vi "Acq_N_Proc.vi"(0 "I2C Ref In":T1={"myRIO Reference"={"myRIO Model"=enum."Unknown", "myRIO Hardware Reference"={"Generic FPGA Reference"=refnum, "Allow multiple opens"=FALSE}}, "I2C Channels Enum"=enum."Not Connected", "I2C Configuration"={"I2C Transfer Rate"=enum."Fast mode (400 kbps)"}}, 1 "Slave_Adress":u8 format="%02o", 2 "I2C Errors":errorcluster, 4 "DIO Ref In":T9, 5 "Int Errors":errorcluster) -> (19 "error IO":errorcluster)   [LabVIEW 2014]
uses:
  <vilib>/myRIO/Instrument Drivers/Onboard IO/DIO/typedefs/DIO Reference.ctl
  <vilib>/myRIO/Common/Instrument Driver Framework/Utilities/typedefs/myRIO Generic Hardware Reference.ctl
  <vilib>/myRIO/Common/Instrument Driver Framework/Utilities/typedefs/Hardware Version Enum.ctl
  <vilib>/myRIO/Common/Instrument Driver Framework/Utilities/typedefs/myRIO v1.0 Reference.ctl
  <vilib>/myRIO/Common/Instrument Driver Framework/Utilities/typedefs/Generic FPGA Reference.ctl
  <vilib>/myRIO/Common/Instrument Driver Framework/myRIO v1.0/DIO/typedefs/DIO Channels List.ctl
  <vilib>/myRIO/Common/Instrument Driver Framework/myRIO v1.0/DIO/typedefs/DIO Channels Enum.ctl
  <vilib>/myRIO/Instrument Drivers/Onboard IO/I2C/typedefs/I2C Reference.ctl
  <vilib>/myRIO/Common/Instrument Driver Framework/myRIO v1.0/I2C/typedefs/I2C Channels Enum.ctl
  <vilib>/myRIO/Instrument Drivers/Onboard IO/I2C/typedefs/I2C Configuration.ctl
  <vilib>/myRIO/Instrument Drivers/Onboard IO/I2C/typedefs/I2C Transfer Rate.ctl
  <vilib>/Platform/TimedLoop/XDataNode/timing_clust.ctl
  <vilib>/Platform/TimedLoop/XDataNode/nitl_modes.ctl
  <vilib>/Platform/TimedLoop/XDataNode/wakeup.ctl
  Globals_Real.vi
  <vilib>/Utility/error.llb/Error Cluster From Error Code.vi
  <vilib>/myRIO/Common/Instrument Driver Framework/myRIO v1.0/DIO/vis/myRIO v1.0 Read DIO.vi
  <vilib>/myRIO/Common/Instrument Driver Framework/myRIO v1.0/I2C/vis/myRIO v1.0 Write I2C.vi
  <vilib>/myRIO/Common/Instrument Driver Framework/myRIO v1.0/I2C/vis/myRIO v1.0 Read I2C.vi
  <vilib>/Platform/TimedLoop/XDataNode/XDataNode.xnode
  <vilib>/Platform/TimedLoop/XDataNode/XDNodeRunTimeDep.lvlib
  <vilib>/myRIO/Instrument Drivers/Onboard IO/DIO/DIO.lvlib
  <vilib>/myRIO/Instrument Drivers/Onboard IO/I2C/I2C.lvlib
panel:
  out "Linear Acceleration [LSB/sec^2]":dbl[](array[numeric])
  out "Angular Displacement (Gyro)":dbl[](array[numeric])
  out "Angular Gyro Rate [LSB/sec]":dbl[](array[numeric])
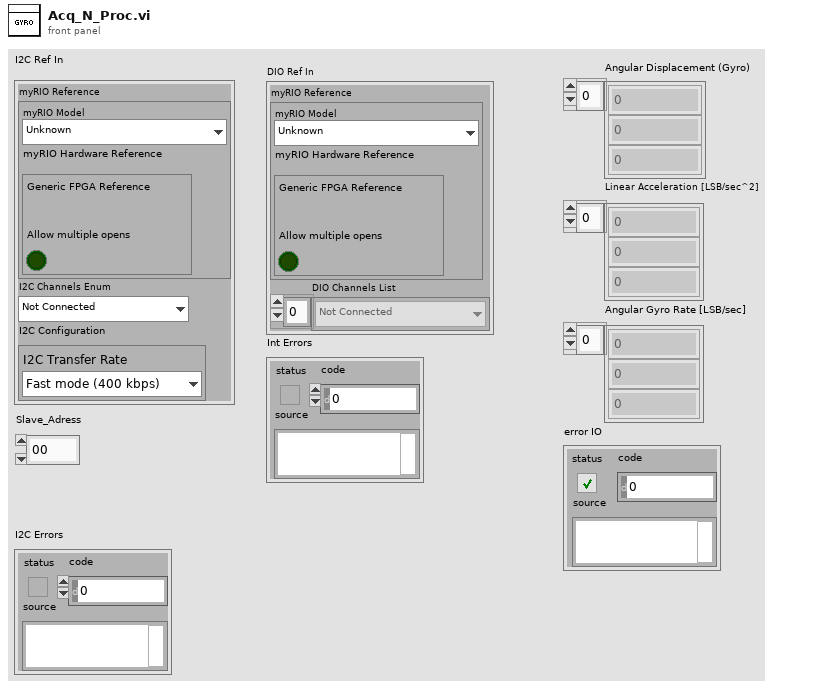
[diagram p1: front panel]
types:
  T1 = typedef "I2C.lvlib/I2C Reference.ctl" = cluster{"myRIO Reference":T2, "I2C Channels Enum":T6, "I2C Configuration":T7}
  T2 = typedef "myRIO Generic Hardware Reference.ctl" = cluster{"myRIO Model":T3, "myRIO Hardware Reference":T4}
  T3 = typedef "Hardware Version Enum.ctl" = enum16{"Unknown", "myRIO-1900", "myRIO-1950"}
  T4 = typedef "myRIO v1.0 Reference.ctl" = cluster{"Generic FPGA Reference":T5, "Allow multiple opens":bool}
  T5 = typedef "Generic FPGA Reference.ctl" = refnum<k20>
  T6 = typedef "I2C Channels Enum.ctl" = enum16{"Not Connected", "A/I2C", "B/I2C"}
  T7 = typedef "I2C.lvlib/I2C Configuration.ctl" = cluster{"I2C Transfer Rate":T8}
  T8 = typedef "I2C.lvlib/I2C Transfer Rate.ctl" = enum16{"Standard mode (100 kbps)", "Fast mode (400 kbps)"}
  T9 = typedef "DIO.lvlib/DIO Reference.ctl" = cluster{"myRIO Reference":T2, "DIO Channels List":T10}
  T10 = typedef "DIO Channels List.ctl" = T11[]
  T11 = typedef "DIO Channels Enum.ctl" = enum16{"Not Connected", "C/DIO0", "C/DIO1", "C/DIO2", "C/DIO3", "C/DIO4", "C/DIO5", "C/DIO6", "C/DIO7", "A/DIO0", "A/DIO1", "A/DIO2", "A/DIO3", "A/DIO4", "A/DIO5", "A/DIO6", "A/DIO7", "A/DIO8", "A/DIO9", "A/DIO10", "A/DIO11", "A/DIO12", "A/DIO13", "A/DIO14", "A/DIO15", "B/DIO0", "B/DIO1", "B/DIO2", "B/DIO3", "B/DIO4", "B/DIO5", "B/DIO6", "B/DIO7", "B/DIO8", "B/DIO9", "B/DIO10", "B/DIO11", "B/DIO12", "B/DIO13", "B/DIO14", "B/DIO15", "LED0", "LED1", "LED2", "LED3", "Button0"}
  T12 = typedef "XDNodeRunTimeDep.lvlib/timing_clust.ctl" = cluster{"Expected End [f-1]":u64, "Actual End [f-1]":u64, "Finished Late? [f-1]":bool, "Expected End [i-1]":u64, "Actual End [i-1]":u64, "Finished Late? [i-1]":bool, "Expected Start [i]":u64, "Actual Start [i]":u64, "Expected Start [f]":u64, "Actual Start [f]":u64, "Source Name":string, "Structure Name":string, "Period":i64, "Deadline":i64, "Offset":i64, "Start":i64, "Priority":i32, "Timeout":i32, "Mode":T13, "Wakeup Reason":T14, "Error":errorcluster, "Source Type":string, "Secondary Source Type":string, "Global End Time":u64, "Global Start Time":u64, "Frame Duration":u64, "Iteration Duration":u64, "Assigned CPU":i32, "I/O Scan Engine Mode":u32}
  T13 = typedef "XDNodeRunTimeDep.lvlib/nitl_modes.ctl" = enum32{"No Change", "Process missed periods, maintain original phase", "Discard missed periods, maintain original phase", "Process missed periods, ignore original phase", "Discard missed periods, ignore original phase"}
  T14 = typedef "XDNodeRunTimeDep.lvlib/wakeup.ctl" = enum32{"Normal", "Aborted", "Asynchronous wakeup", "Timing source error", "Timed loop error", "Timeout"}
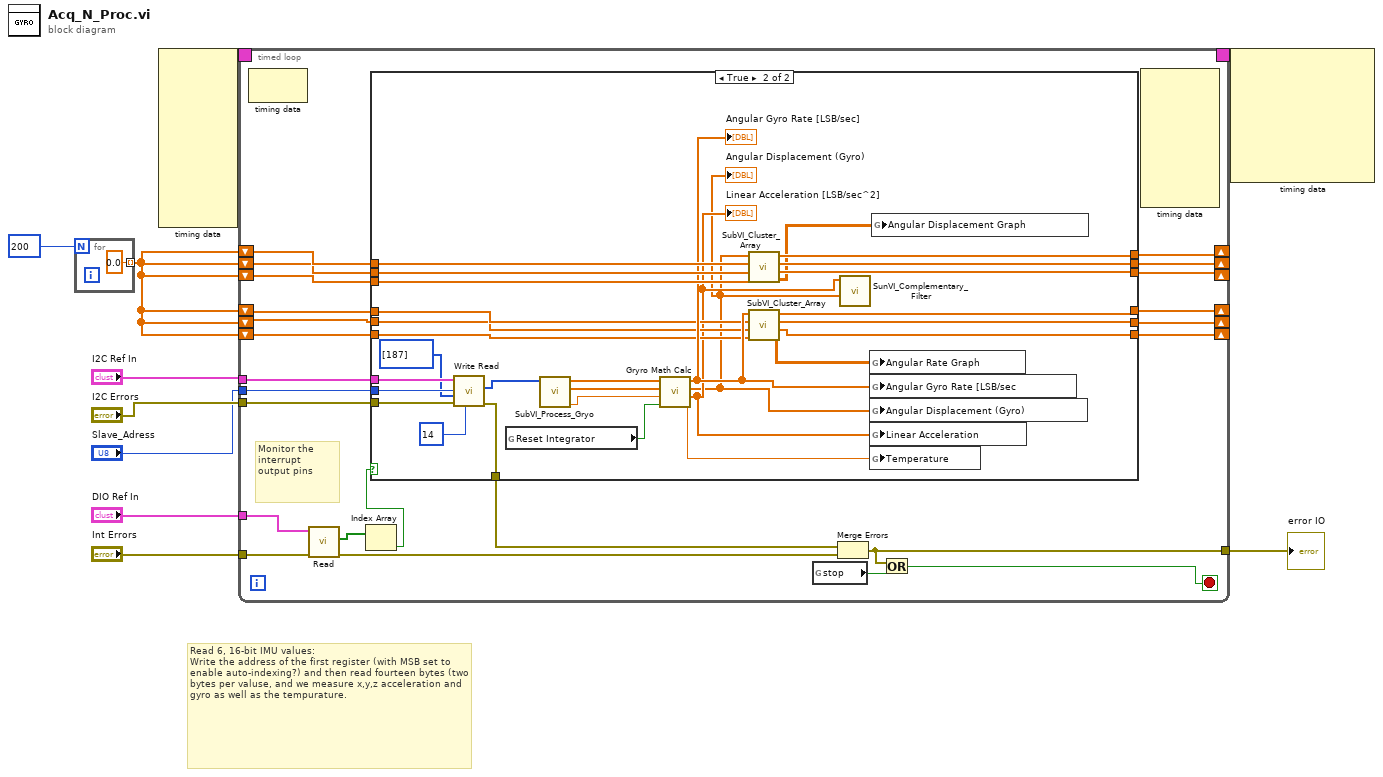
[diagram p0: block diagram]
diagram:
  # "Read 6, 16-bit IMU values:\nWrite the address of the first register (with MSB set to enable auto-indexing?) and then read fourteen bytes (two bytes per valuse, and we measure x,y,z acceleration and gyro as well as the tempurature."
  n1 = for {
    N: 200 -> [_]
    tunnel: [0.0] -> w1 mode=indexing
  }
  n2 = node-c288() -> (w10:T12)  [unwired: 10 in]
  n3 = timed-loop {
    timing: w10 -> [_]
    timing-out: [_] -> w9
    tunnel: "DIO Ref In" -> [w35]
    tunnel: "Int Errors" -> [w34]
    tunnel: "I2C Ref In" -> [w28]
    tunnel: "I2C Errors" -> [w27]
    tunnel: "Slave_Adress" -> [w26]
    tunnel: [w24] -> w3
    shift-right: [w22] -> _
    shift-left: w1 -> [w23]
    shift-right: [w19] -> _
    shift-left: w1 -> [w21]
    shift-right: [w18] -> _
    shift-left: w1 -> [w20]
    shift-right: [w14] -> _
    shift-left: w1 -> [w17]
    shift-right: [w13] -> _
    shift-left: w1 -> [w16]
    shift-right: [w12] -> _
    shift-left: w1 -> [w15]
    stop <- w29 stop-if-true
    # "Monitor the\ninterrupt\noutput pins"
    n4 = node-c288() -> ()  [unwired: 1 in, 1 out]
    n5 = call <vilib>:"Read.vi"("error in (no error)"=w34, "DIO Ref In"=w35) -> ("error out"=w32:errorcluster, "Values"=w33:bool[])  [unwired: 7 in, 1 out]
    n6 = Index Array(array=w33) -> (element=w31:bool)  [unwired: 1 in]
    n7 = case shown="True" w31 {
      tunnel: w28 -> [_ w71]
      tunnel: w27 -> [w42 w67]
      tunnel: w26 -> [_ w70]
      tunnel: [w42 w68] -> w25
      tunnel: w23 -> [w41 w59]
      tunnel: [w41 w55] -> w22
      tunnel: w21 -> [w40 w58]
      tunnel: w20 -> [w39 w57]
      tunnel: [w40 w54] -> w19
      tunnel: [w39 w56] -> w18
      tunnel: w17 -> [w38 w51]
      tunnel: w16 -> [w37 w50]
      tunnel: w15 -> [w36 w49]
      tunnel: [w38 w48] -> w14
      tunnel: [w37 w47] -> w13
      tunnel: [w36 w46] -> w12
      frame False {
      }
      frame True {
        n8 = call <vilib>:"Write Read.vi"("Byte Count"=u32 14, "error in (no error)"=w67, "Bytes to Write"=u8[] [187], "Slave Address (7-bit)"=w70, "I2C Ref In"=w71) -> ("error out"=w68:errorcluster, "Bytes Read"=w65:u8[])  [unwired: 3 in, 1 out]
        n9 = global read "Globals_Real.vi" "Reset Integrator"() -> (w63:bool)
        n10 = call "SubVI_Process_Gryo.vi"("Bytes Read"=w65) -> ("Temperature (Pure doule precision HW)"=w64:dbl, "Gyroscopic Rate precision"=w60:dbl[], "Acceleration Rate precision float"=w61:dbl[])  [unwired: 8 in]
        n11 = call "Gryro Math Calc.vi"("Reset Integrator"=w63, "Temperature (Pure doule precision HW) in"=w64, "Gyroscopic Cluster Values In"=w60, "Accel Array"=w61) -> ("Temperature (Scaled) out"=w62:dbl, "Linear Acceleration [LSB/sec^2]"=w44:dbl[], "Angular Displacement (Gyro)"=w43:dbl[], "Angular Gyro Rate [LSB/sec]"=w52:dbl[])  [unwired: 4 in]
        "Angular Gyro Rate [LSB/sec]" <- w52
        "Angular Displacement (Gyro)" <- w43
        "Linear Acceleration [LSB/sec^2]" <- w44
        n12 = call "SubVI_Cluster_Array.vi"("Z Array in"=w57, "Y Array in"=w58, "X Array in"=w59, "Angular Displacement Feedback (Gyro)"=w43) -> ("Appended array"=w53:dbl[][], "Z Out"=w56:dbl[], "Y Out"=w54:dbl[], "X Out"=w55:dbl[])  [unwired: 4 in]
        n13 = call "SubVI_Cluster_Array.vi"("Z Array in"=w49, "Y Array in"=w50, "X Array in"=w51, "Angular Displacement Feedback (Gyro)"=w52) -> ("Appended array"=w45:dbl[][], "Z Out"=w46:dbl[], "Y Out"=w47:dbl[], "X Out"=w48:dbl[])  [unwired: 4 in]
        n14 = call "SunVI_Complementary_Filter.vi"("Gryo Displacement"=w43, "Linear Acceleration"=w44) -> ()  [unwired: 10 in]
        n15 = global write "Globals_Real.vi" "Angular Rate Graph"(w45) -> ()
        n16 = global write "Globals_Real.vi" "Angular Gyro Rate [LSB/sec"(w52) -> ()
        n17 = global write "Globals_Real.vi" "Angular Displacement (Gyro)"(w43) -> ()
        n18 = global write "Globals_Real.vi" "Linear Acceleration"(w44) -> ()
        n19 = global write "Globals_Real.vi" "Temperature"(w62) -> ()
        n20 = global write "Globals_Real.vi" "Angular Displacement Graph"(w53) -> ()
      }
    }
    n21 = global read "Globals_Real.vi" "stop"() -> (w30:bool)
    n22 = Merge Errors "Merge Errors"(w25, w32) -> (w24:errorcluster)
    n23 = Or(x=w24, y=w30) -> (x .or. y?=w29:bool)
    n24 = node-c288() -> ()  [unwired: 8 in, 1 out]
  }
  "error IO" <- w3
  n25 = node-c288(w9) -> ()  [unwired: 7 out]
